vi "Read URL.vi"(8 "error in (no error)":errorcluster, 11 "WebView2 Control in":refnum<class "WebView2 Control.lvclass">) -> (0 "error out":errorcluster, 2 "Source":string, 3 "WebView2 Control out":refnum<class "WebView2 Control.lvclass">)   [LabVIEW 2020, in "WebView2.lvlib" / "WebView2 Control.lvclass"]
uses:
  WebView2 Control.lvclass
  WebView2 Control.lvclass/WebView2 Control.ctl
  C:/Users/Simon/Documents/GitHub/LV-WebView2/Source/Libs/Microsoft.Web.WebView2.Core.dll
  Libs/Microsoft.Web.WebView2.Core.dll
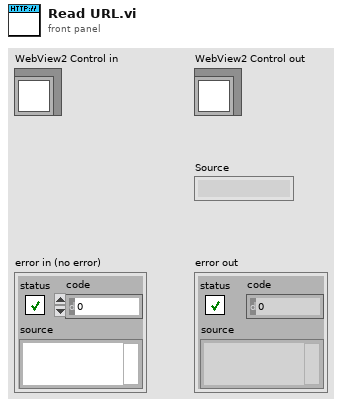
[diagram p1: front panel]
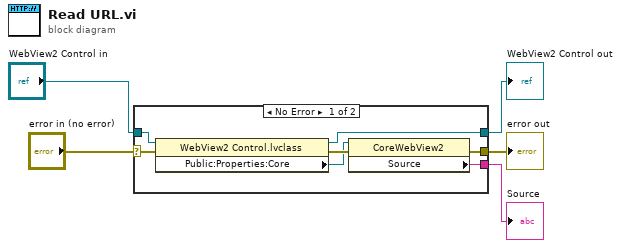
[diagram p0: block diagram]
diagram:
  n1 = case shown="No Error" "error in (no error)" {
    selector: "error in (no error)" -> [w12 w14]
    tunnel: [w8 w14] -> w4
    tunnel: [w9 w13] -> w2
    tunnel: "WebView2 Control in" -> [w10 w13]
    tunnel: [w6 _] -> w1
    frame No Error {
      n2 = property class="WebView2 Control.lvclass"(reference=w10, error in=w12) -> (reference out=w9:refnum<class "WebView2 Control.lvclass">, error out=w11:errorcluster, "Public:Properties:Core"=w7:refnum<k24>)
      n3 = property class="CoreWebView2"(reference=w7, error in=w11) -> (error out=w8:errorcluster, "Source"=w6:string)  [unwired: 1 out]
    }
    frame Error {
    }
  }
  "error out" <- w4
  "WebView2 Control out" <- w2
  "Source" <- w1
